vi "auto.vi"() -> ()   [LabVIEW 2016]
uses:
  Robot Global Data.vi
  <vilib>/Rock Robotics/Network Tables/NT Read Number.vi
  <vilib>/addons/control/pid/pid.llb/PID (DBL).vi
  <vilib>/addons/control/pid/NI_PID_pid.lvlib
panel:
  in  "PID gains":T1={"proportional gain (Kc)"=0.015, "integral time (Ti, min)"=0.0, "derivative time (Td, min)"=0.0} {"derivative time (Td, min)" format="%.3f"; "integral time (Ti, min)" format="%.3f"; "proportional gain (Kc)" format="%.3f"}
  in  "y":dbl
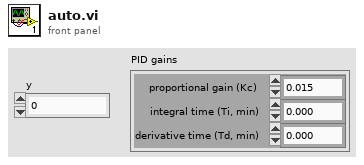
[diagram p1: front panel]
types:
  T1 = cluster{"proportional gain (Kc)":dbl, "integral time (Ti, min)":dbl, "derivative time (Td, min)":dbl}
  T2 = typedef "WPI_EncoderDevRef.ctl" = cluster{"DevStatus":errorcluster, "EncoderIndex":T3, "CounterIndex":T4, "DistancePerCount":dbl, "Decoding Type":T5}
  T3 = typedef "FPGA_EncoderIdx.ctl" = enum8{"Enc 0", "Enc 1", "Enc 2", "Enc 3", "Enc 4", "Enc 5", "Enc 6", "Enc 7", "Invalid"}
  T4 = typedef "FPGA_CounterCtrSystemIndex.ctl" = enum8{"Ctr 0", "Ctr 1", "Ctr 2", "Ctr 3", "Ctr 4", "Ctr 5", "Ctr 6", "Ctr 7", "Invalid"}
  T5 = typedef "WPI_EncoderType.ctl" = enum16{"1x", "2x", "4x"}
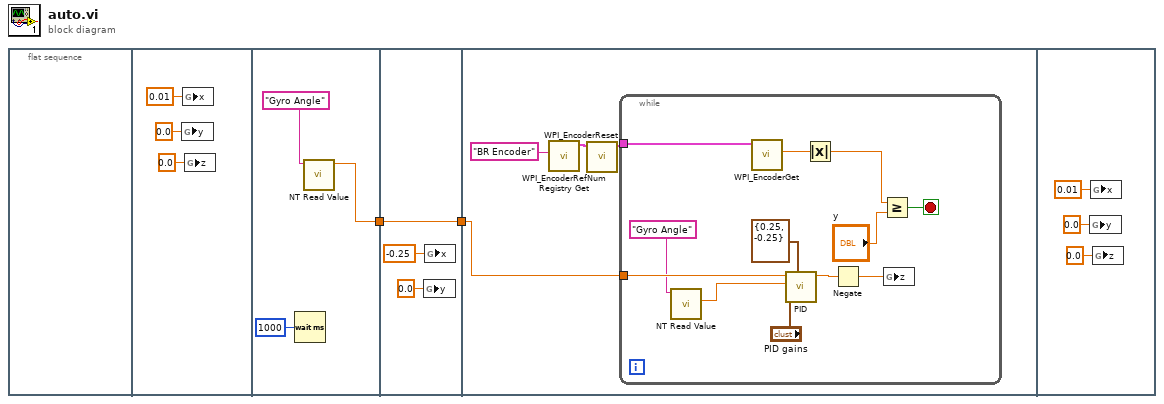
[diagram p0: block diagram]
diagram:
  n1 = flat-sequence {
    tunnel: [w6] -> w2
    tunnel: w2 -> [w9]
    tunnel: [w9] -> w1
    tunnel: w1 -> [w12]
    frame #0 {
    }
    frame #1 {
      n2 = global write "Robot Global Data.vi" "y"(0.0 ("y")) -> ()
      n3 = global write "Robot Global Data.vi" "x"(0.01 ("x")) -> ()
      n4 = global write "Robot Global Data.vi" "z"(0.0 ("z")) -> ()
    }
    frame #2 {
      n5 = Wait (ms)(milliseconds to wait=u32 1000) -> ()  [unwired: 1 out]
      n6 = call-poly <vilib>:"NT Read Value.vi"("Name"="Gyro Angle") -> ("Numeric"=w6:dbl)  [unwired: 9 in, 1 out]
    }
    frame #3 {
      n7 = global write "Robot Global Data.vi" "y"(0.0 ("y")) -> ()
      n8 = global write "Robot Global Data.vi" "x"(-0.25 ("x")) -> ()
    }
    frame #4 {
      n9 = call <vilib>:"WPI_EncoderRefNum Registry Get.vi"("refnum name"="BR Encoder") -> ("EncoderDevRef"=w14:T2)  [unwired: 9 in, 1 out]
      n10 = call <vilib>:"WPI_EncoderReset.vi"("EncoderDevRef"=w14) -> ("EncoderDevRef"=w13:T2)  [unwired: 9 in, 1 out]
      n11 = while {
        tunnel: w13 -> [w27]
        tunnel: w12 -> [w21]
        stop <- w25 stop-if-true
        n12 = call-poly <vilib>:"NT Read Value.vi"("Name"="Gyro Angle") -> ("Numeric"=w19:dbl)  [unwired: 9 in, 1 out]
        n13 = call <vilib>:"WPI_EncoderGet.vi"("EncoderDevRef"=w27) -> ("Distance"=w26:dbl)  [unwired: 5 in, 5 out]
        n14 = call-poly <vilib>:"PID.vi"("output range"=cluster{"output high":dbl, "output low":dbl} {"output high"=0.25, "output low"=-0.25}, "PID gains"="PID gains", "process variable"=w19, "setpoint"=w21) -> ("output"=w23:dbl)  [unwired: 6 in, 1 out]
        n15 = Absolute Value(x=w26) -> (abs(x)=w17:dbl)
        n16 = Negate(x=w23) -> (-x=w18:dbl)
        n17 = Greater Or Equal?(x=w17, y="y") -> (x >= y?=w25:bool)
        n18 = global write "Robot Global Data.vi" "z"(w18) -> ()
      }
    }
    frame #5 {
      n19 = global write "Robot Global Data.vi" "y"(0.0 ("y")) -> ()
      n20 = global write "Robot Global Data.vi" "x"(0.01 ("x")) -> ()
      n21 = global write "Robot Global Data.vi" "z"(0.0 ("z")) -> ()
    }
  }
